vi "User Interferece_1.vi"() -> ()   [LabVIEW 2022 SP3]
panel:
  out "Parola Out":string
  out "Kulanici Out":string
  in  "Parola":string
  in  "Kulanici Adi":string
  in  "stop":bool
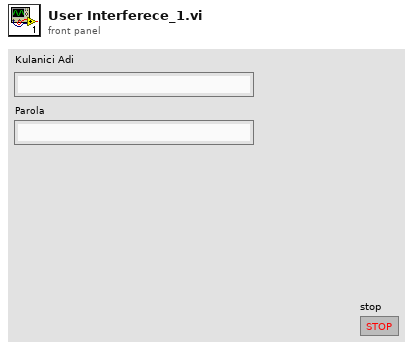
[diagram p1: front panel]
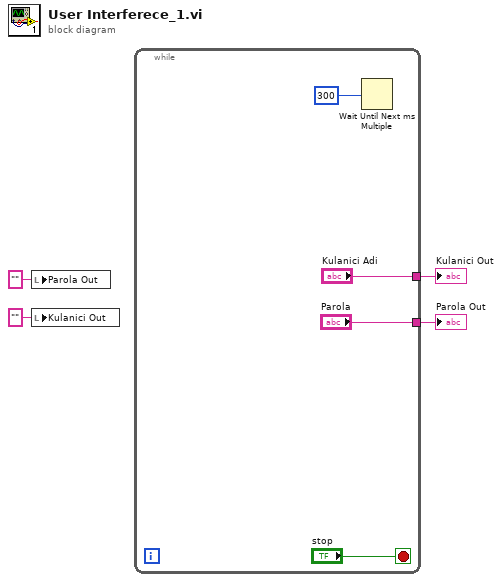
[diagram p0: block diagram]
diagram:
  n1 = local write "Parola Out"("" ("Parola Out")) -> ()
  n2 = local write "Kulanici Out"("" ("Kulanici Out")) -> ()
  n3 = while {
    tunnel: ["Parola"] -> w4
    tunnel: ["Kulanici Adi"] -> w3
    stop <- "stop" stop-if-true
    n4 = Wait Until Next ms Multiple(millisecond multiple=u32 300 ("millisecond timer value")) -> ()  [unwired: 1 out]
  }
  "Kulanici Out" <- w3
  "Parola Out" <- w4
